vi "Stop Core.vi"(10 "final error code":i32, 11 "Server in":refnum<class "Server.lvclass">) -> (3 "Server out":refnum<class "Server.lvclass">)   [LabVIEW 2014, in "Server.lvlib" / "Server.lvclass"]
doc: "(<B>Filename</B>: Actor Framework.lvlib:Actor.lvclass:Stop Core.vi)\n\nDefines what the actor does before it stops. Use the <B>final error code</B> input to determine whether the actor shut down in response to an error.\n\nBy default, this method passes the Stop message along to all auto-stop nested actors. A descendant class may override this method to define additional behavior, such as shutting down any processes the actor initiated in its override of the Actor Core method."
uses:
  Server.lvclass
  <vilib>/ActorFramework/Actor/Actor.lvclass
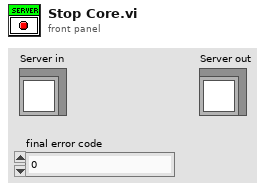
[diagram p1: front panel]
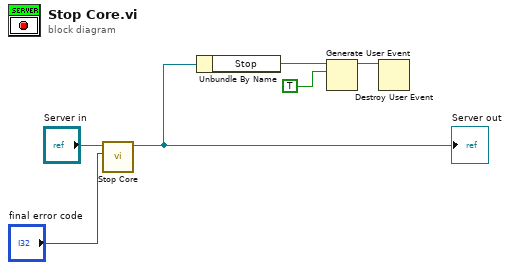
[diagram p0: block diagram]
diagram:
  n1 = call-parent "Stop Core.vi"("final error code"="final error code", "Actor in"="Server in") -> ("Actor out"=w4:refnum<class "Server.lvclass">)  [unwired: 9 in]
  "Server out" <- w4
  n2 = Unbundle By Name(w4) -> ("Stop"=w3:refnum<user-event>)
  n3 = Generate User Event(user event=w3, event data cluster=TRUE) -> (user event out=w1:refnum<user-event>)  [unwired: 2 in, 1 out]
  n4 = Destroy User Event(user event=w1) -> ()  [unwired: 1 in, 1 out]
